vi "Generate Signal.vi"(8 "error in (no error)":errorcluster, 9 "Amplitude (1)":dbl=1.0, 10 "Frequency (1000 Hz)":dbl=1000.0, 11 "Simulated Function Generator in":refnum<class "Simulated Function Generator.lvclass">) -> (0 "error out":errorcluster, 3 "Simulated Function Generator out":refnum<class "Simulated Function Generator.lvclass">)   [LabVIEW 2018, in "Simulated Function Generator.lvclass"]
uses:
  Simulated Function Generator.lvclass
  Common Components/Hardware/FGEN/Function Generator.lvclass
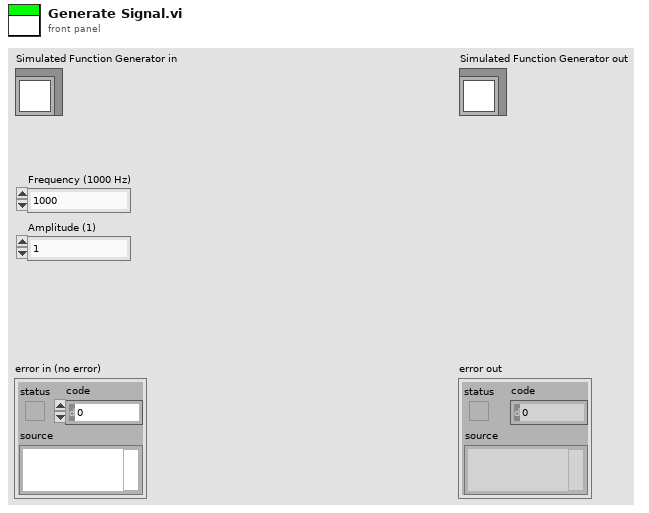
[diagram p1: front panel]
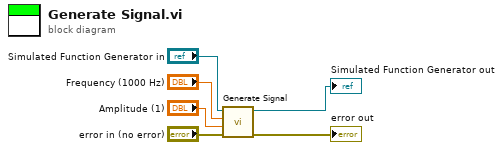
[diagram p0: block diagram]
diagram:
  n1 = call-parent "Generate Signal.vi"("error in (no error)"="error in (no error)", 9:"Amplitude (1)", "Frequency (1000 Hz)"="Frequency (1000 Hz)", "Function Generator in"="Simulated Function Generator in") -> ("error out"=→"error out":errorcluster, "Function Generator out"=→"Simulated Function Generator out":refnum<class "Simulated Function Generator.lvclass">)  [unwired: 6 in]
